vi "Export Parameters to Clipboard Wrapper.vi"(8 "error in (no error)":errorcluster) -> (0 "error out":errorcluster)   [LabVIEW 2019]
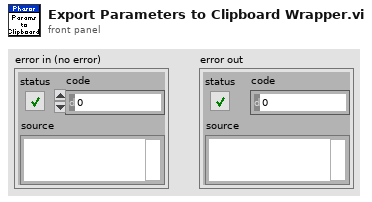
[diagram p1: front panel]
types:
  T1 = typedef "SEPL Parameters.ctl" = cluster{"Display Parameters":T2, "Phasor Parameters":T4, "Decay & IRF Parameters":T7, "Gate Parameters":T9, "Detector Parameters":T12}
  T2 = typedef "Phasor Explorer Display Parameters.ctl" = cluster{"# Points":i32, "Ramp Type":enum16{"Linear", "Logarithmic"}, "Type of Series":T3, "Min tau":dbl[unit], "Max tau":dbl[unit], "Include 0":bool, "Include Infinity":bool}
  T3 = typedef "Type of Series.ctl" = enum16{"1-Exp Decays", "Linear Combination of 1-Exp"}
  T4 = typedef "Phasor Explorer Phasor Parameters.ctl" = cluster{"Harmonic Frequency":dbl[unit], "Use f* = 1/D Frequency":bool, "Calibrated Phasor":bool, "Calibration Lifetime":dbl[unit], "Phasor Calculation":T5, "SEPL Type":T6, "# Gates":dbl, "Square Gate Width":dbl[unit], "Show Ticks":bool}
  T5 = typedef "Phasor Calculation Type.ctl" = enum16{"Direct Sum", "Analytical Formula"}
  T6 = typedef "SEPL Type.ctl" = enum16{"UC", "L_N", "L_N[W]", "L_X"}
  T7 = typedef "Phasor Explorer Decay Parameters.ctl" = cluster{"Lifetime":dbl[unit], "IRF Offset":dbl[unit], "IRF Period":dbl[unit], "Normalized Decays":bool, "IRF Model":T8, "IRF Parameter 1":dbl[unit]}
  T8 = typedef "IRF Model.ctl" = enum16{"Dirac", "Exponential"}
  T9 = typedef "Phasor Explorer Gate Parameters.ctl" = cluster{"First Gate Start":dbl[unit], "Use Gate Center":bool, "Gate Width":dbl[unit], "Gate Step":dbl[unit], "# Gates":dbl, "Gate Type":T10, "Edge Width":dbl[unit], "Top Slope":dbl[unit], "Reversed Sawtooth?":bool, "Analytical Computation":bool, "Integration":enum32{"Item 0", "Item 1"}, "Tolerance":dbl, "# Steps":dbl, "Type of User-defined Function":T11, "Use Gate Step":bool}
  T10 = typedef "Gate Type.ctl" = enum16{"Square", "Finite Edge Square", "Finite Edge, Tilted Top Square", "Triangle", "Sawtooth", "User-defined"}
  T11 = typedef "Type of User-defined Function.ctl" = enum16{"Gate", "IRF"}
  T12 = typedef "Phasor Explorer Detector Parameters.ctl" = cluster{"Frames/Image":i32, "Gates/Frame":i32, "Bits/Frame":i32, "Multiplicity":i32, "Incident Signal":dbl, "Poisson Signal":bool}
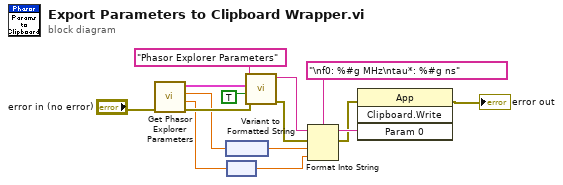
[diagram p0: block diagram]
diagram:
  n1 = call "Get Phasor Explorer Parameters.vi"("Error In"="error in (no error)") -> ("Error Out"=w4:errorcluster, "tau*"=w2:dbl[unit], "f0"=w3:dbl[unit], "Phasor Explorer Parameters"=w5:T1)  [unwired: 7 in]
  n2 = node(w3) -> (w9:dbl)
  n3 = node(w2) -> (w8:dbl)
  n4 = call "Variant to Formatted String.vi"("Error In"=w4, "Hide Long Cluster Names (T)"=TRUE ("Hide Long Names (Cluster)"), "Variant"=w5, "Label"="Phasor Explorer Parameters" ("Label.Text")) -> ("Error Out"=w10:errorcluster, "String"=w14:string)  [unwired: 6 in]
  n5 = Format Into String(format string="\nf0: %#g MHz\ntau*: %#g ns", initial string=w14, error in=w10, w9, w8) -> (resulting string=w13:string, error out=w11:errorcluster)
  n6 = invoke class="App" method="Clipboard.Write"(error in=w11, "Param 0"=w13) -> (error out=→"error out":errorcluster)  [unwired: 2 in, 3 out]
